vi "Auton-InterpretDataString.vi"() -> ()   [LabVIEW 2014]
uses:
  <vilib>/Rock Robotics/Network Tables/SD Read String.vi
panel:
  out "Success Array":bool[](array[boolean])
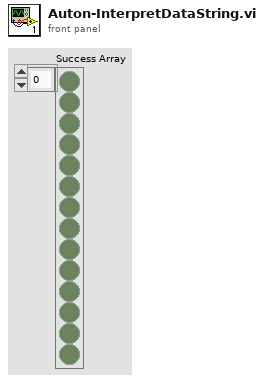
[diagram p1: front panel]
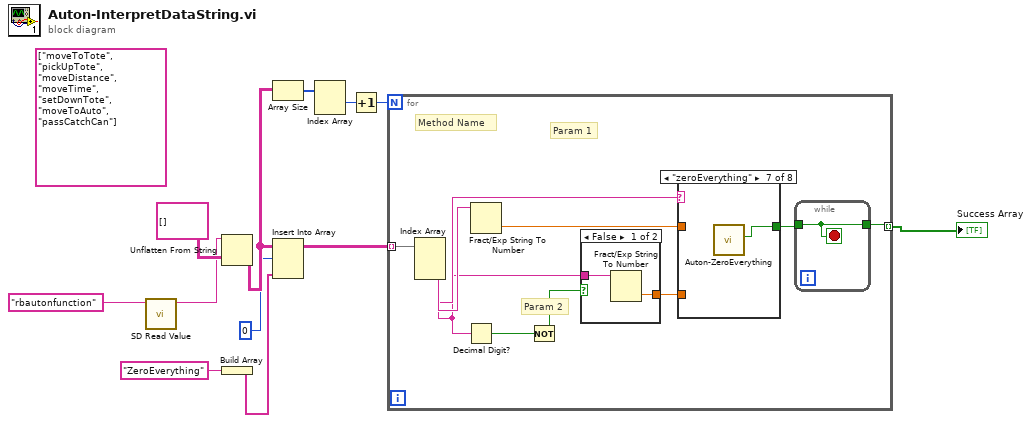
[diagram p0: block diagram]
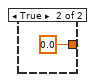
[diagram p2: hidden frame]
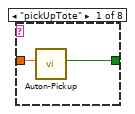
[diagram p3: hidden frame]
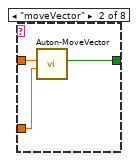
[diagram p4: hidden frame]
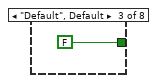
[diagram p5: hidden frame]
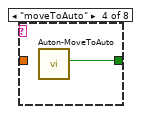
[diagram p6: hidden frame]
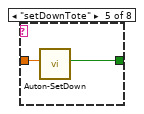
[diagram p7: hidden frame]
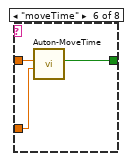
[diagram p8: hidden frame]
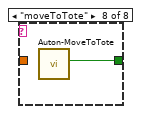
[diagram p9: hidden frame]
diagram:
  (unwired) string[] ["moveToTote", "pickUpTote", "moveDistance", "moveTime", "setDownTote", "moveToAuto", "passCatchCan"] ("string array")
  n1 = call-poly <vilib>:"SD Read Value.vi"("Name"="rbautonfunction") -> ("String"=w10:string)  [unwired: 8 in, 2 out]
  n2 = Unflatten From String(type=string[][] [], binary string=w10) -> (value=w5:string[][])  [unwired: 3 in, 2 out]
  n3 = Build Array("ZeroEverything") -> (w3:string[])
  n4 = Array Size(array=w5) -> (size(s)=w9:i32[])
  n5 = Insert Into Array(array=w5, index (row)=0, new element=w3) -> (w2:string[][])  [unwired: 1 in]
  n6 = Index Array(array=w9) -> (element #1=w7:i32)  [unwired: 2 in, 1 out]
  n7 = Increment(x=w7) -> (x+1=w1:i32)
  n8 = for {
    N: w1 -> [_]
    tunnel: w2 -> [w22] mode=indexing
    tunnel: [w13] -> w8 mode=indexing
    # "Param 2"
    # "Param 1"
    # "Method Name"
    n9 = Index Array(array=w22) -> (element #1=w20:string, element #2=w21:string, element #3=w18:string)  [unwired: 3 in]
    n10 = Decimal Digit?(1:w18) -> (0:w16:bool)
    n11 = Fract/Exp String To Number(string=w21) -> (number=w19:dbl)  [unwired: 3 in, 1 out]
    n12 = Not(x=w16) -> (.not. x?=w17:bool)
    n13 = case shown="False" w17 {
      tunnel: w18 -> [w25 _]
      tunnel: [w24 0.0] -> w15
      frame False {
        n14 = Fract/Exp String To Number(string=w25) -> (number=w24:dbl)  [unwired: 3 in, 1 out]
      }
      frame True {
      }
    }
    n15 = case shown="\"zeroEverything\"" w20 {
      tunnel: [w28 w30 FALSE w33 w35 w38 w39 w40] -> w14
      tunnel: w19 -> [w27 w31 _ _ w34 w37 _ _]
      tunnel: w15 -> [_ w29 _ _ _ w36 _ _]
      frame "pickUpTote" {
        n16 = call "Auton-Pickup.vi"("ToHeight"=w27) -> ("Done"=w28:bool)  [unwired: 10 in]
      }
      frame "moveVector" {
        n17 = call "Auton-MoveVector.vi"("Angle"=w29, "Distance"=w31) -> ("Done?"=w30:bool)  [unwired: 9 in]
      }
      frame "Default", Default {
      }
      frame "moveToAuto" {
        n18 = call "Auton-MoveToAuto.vi"() -> ("Boolean"=w33:bool)  [unwired: 11 in]
      }
      frame "setDownTote" {
        n19 = call "Auton-SetDown.vi"("OnTopOf"=w34) -> ("Done"=w35:bool)  [unwired: 10 in]
      }
      frame "moveTime" {
        n20 = call "Auton-MoveTime.vi"("Param 2"=w36, "Param 1"=w37) -> ("Done"=w38:bool)  [unwired: 9 in]
      }
      frame "zeroEverything" {
        n21 = call "Auton-ZeroEverything.vi"() -> ("Done?"=w39:bool)  [unwired: 11 in]
      }
      frame "moveToTote" {
        n22 = call "Auton-MoveToTote.vi"() -> ("Task Complete"=w40:bool)  [unwired: 11 in]
      }
    }
    n23 = while {
      tunnel: w14 -> [w23]
      tunnel: [w23] -> w13
      stop <- w23 stop-if-true
    }
  }
  "Success Array" <- w8
